vi "Merge Sort Transposed Time Series Data.vi"(0 "Time Series Array A":dbl[][](array[numeric]), 1 "Ignore Duplicates? (F)":bool, 3 "Time Series Array B":dbl[][](array[numeric])) -> (6 "Sorted Time Series Array":dbl[][](array[numeric]))   [LabVIEW 2013, in "Data Log Fetcher.lvlib"]
uses:
  Data Log Fetcher.lvlib
panel:
  out "A Index":i32
  out "B Index":i32
  out "B Count":i32
  out "A Count":i32
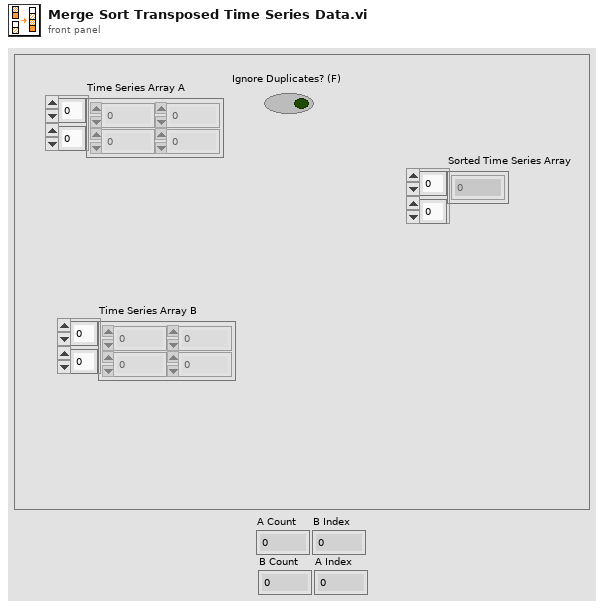
[diagram p1: front panel]
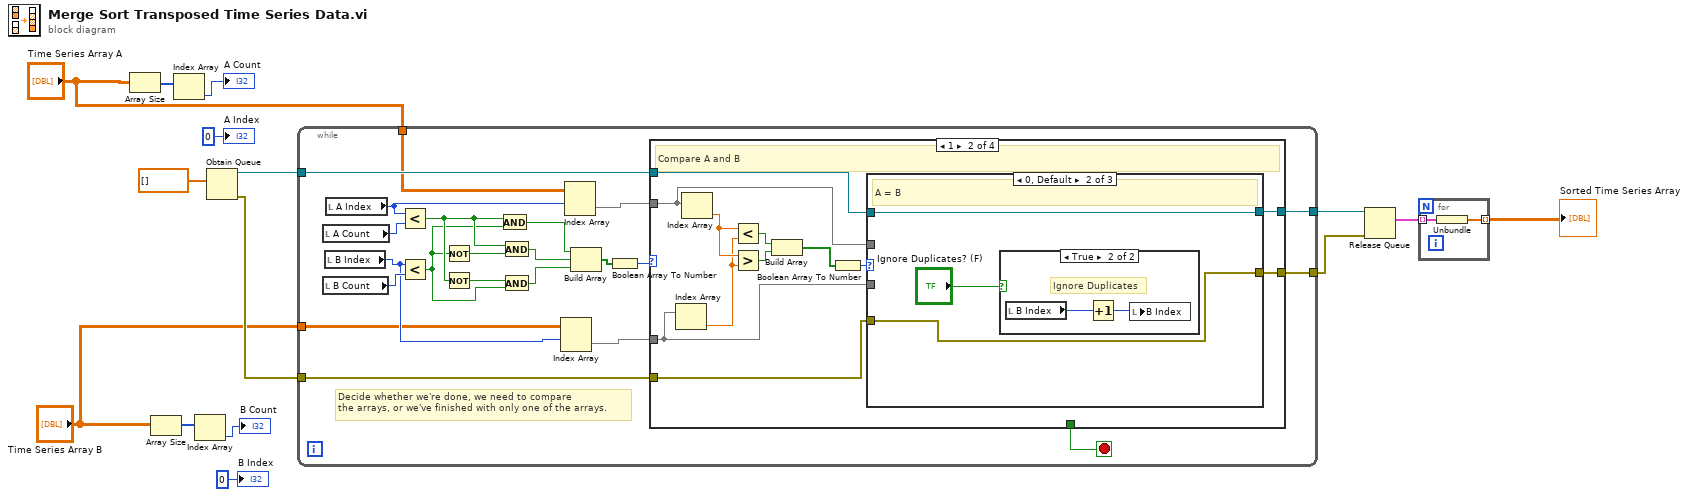
[diagram p0: block diagram]
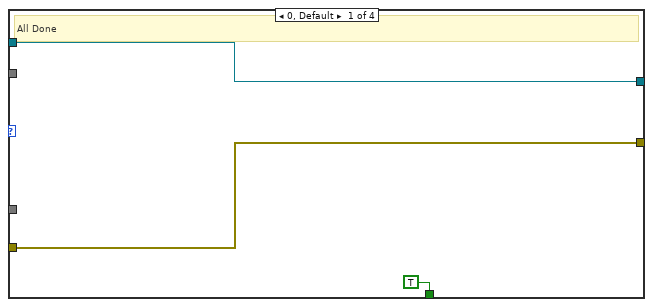
[diagram p2: hidden frame]
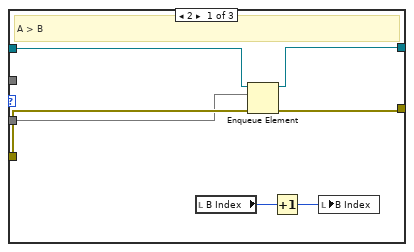
[diagram p3: hidden frame]
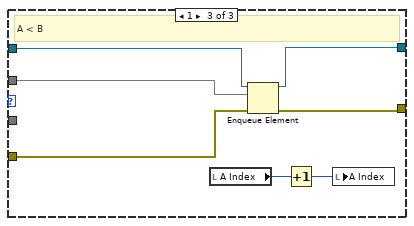
[diagram p5: hidden frame]
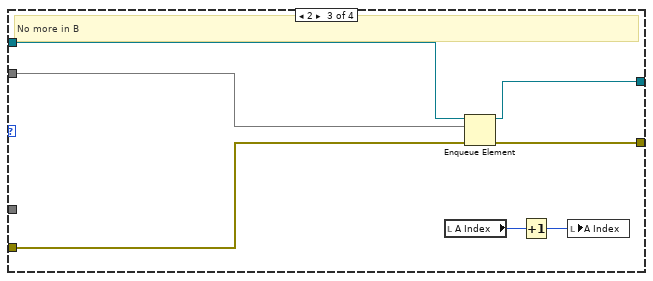
[diagram p6: hidden frame]
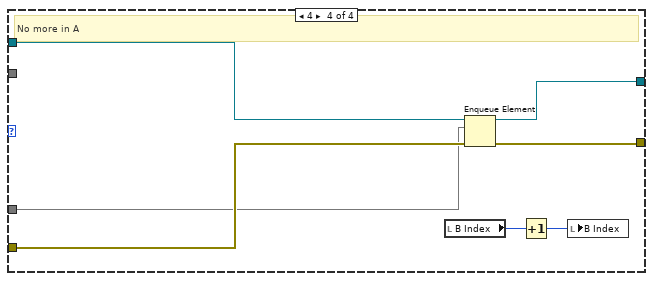
[diagram p7: hidden frame]
diagram:
  n1 = Array Size(array="Time Series Array A") -> (size(s)=w8:i32[])
  n2 = Array Size(array="Time Series Array B") -> (size(s)=w6:i32[])
  n3 = Index Array(array=w8) -> (element=→"A Count":i32)  [unwired: 1 in]
  n4 = Index Array(array=w6) -> (element=→"B Count":i32)  [unwired: 1 in]
  n5 = Obtain Queue(element data type=dbl[] []) -> (queue out=w14:refnum<queue>, error out=w13:errorcluster)  [unwired: 4 in, 1 out]
  n6 = while {
    tunnel: w14 -> [w26]
    tunnel: [w25] -> w10
    tunnel: [w24] -> w15
    tunnel: w13 -> [w23]
    tunnel: "Time Series Array A" -> [w17]
    tunnel: "Time Series Array B" -> [w16]
    stop <- w18 stop-if-true
    # "Decide whether we're done, we need to compare\nthe arrays, or we've finished with only one of the arrays."
    n7 = local read "A Count"() -> (w37:i32)
    n8 = local read "B Count"() -> (w36:i32)
    n9 = local read "B Index"() -> (w21:i32)
    n10 = local read "A Index"() -> (w22:i32)
    n11 = Less?(x=w22, y=w37) -> (x < y?=w33:bool)
    n12 = Less?(x=w21, y=w36) -> (x < y?=w32:bool)
    n13 = Not(x=w32) -> (.not. x?=w30:bool)
    n14 = Not(x=w33) -> (.not. x?=w29:bool)
    n15 = And(x=w33, y=w32) -> (x .and. y?=w35:bool)
    n16 = And(x=w33, y=w30) -> (x .and. y?=w34:bool)
    n17 = And(x=w29, y=w32) -> (x .and. y?=w31:bool)
    n18 = Index Array(array=w16, index (row)=w21) -> (element=w20:dbl[])  [unwired: 1 in]
    n19 = Index Array(array=w17, index (row)=w22) -> (element=w19:dbl[])  [unwired: 1 in]
    n20 = Build Array(w35, w34, w31) -> (w28:bool[])
    n21 = Boolean Array To Number(Boolean array=w28) -> (number=w27:u32)
    n22 = case shown="1" w27 {
      tunnel: w26 -> [w40 w52 w78 w85]
      tunnel: w19 -> [_ w44 w76 _]
      tunnel: w20 -> [_ w42 _ w83]
      tunnel: w23 -> [w39 w45 w77 w84]
      tunnel: [w39 w51 w74 w81] -> w25
      tunnel: [w40 w50 w75 w82] -> w24
      tunnel: [TRUE _ _ _] -> w18
      frame 0, Default {
        # "All Done"
      }
      frame 1 {
        # "Compare A and B"
        n23 = Index Array(array=w42) -> (element=w41:dbl)  [unwired: 1 in]
        n24 = Index Array(array=w44) -> (element=w43:dbl)  [unwired: 1 in]
        n25 = Less?(x=w43, y=w41) -> (x < y?=w49:bool)
        n26 = Greater?(x=w43, y=w41) -> (0:w48:bool)
        n27 = Build Array(w49, w48) -> (w47:bool[])
        n28 = Boolean Array To Number(Boolean array=w47) -> (number=w46:u32)
        n29 = case shown="0, Default" w46 {
          tunnel: w52 -> [w59 w60 w71]
          tunnel: w44 -> [_ _ w70]
          tunnel: w42 -> [w53 _ _]
          tunnel: w45 -> [w58 w61 w69]
          tunnel: [w56 w61 w67] -> w51
          tunnel: [w57 w60 w68] -> w50
          frame 2 {
            # "A > B"
            n30 = local read "B Index"() -> (w54:i32)
            n31 = Enqueue Element(queue=w59, element=w53, error in (no error)=w58) -> (queue out=w57:refnum<queue>, error out=w56:errorcluster)  [unwired: 1 in, 1 out]
            n32 = Increment(x=w54) -> (x+1=w55:i32)
            n33 = local write "B Index"(w55) -> ()
          }
          frame 0, Default {
            # "A = B"
            n34 = case shown="True" "Ignore Duplicates? (F)" {
              frame False {
              }
              frame True {
                # "Ignore Duplicates"
                n35 = local read "B Index"() -> (w64:i32)
                n36 = Increment(x=w64) -> (x+1=w63:i32)
                n37 = local write "B Index"(w63) -> ()
              }
            }
          }
          frame 1 {
            # "A < B"
            n38 = local read "A Index"() -> (w65:i32)
            n39 = Enqueue Element(queue=w71, element=w70, error in (no error)=w69) -> (queue out=w68:refnum<queue>, error out=w67:errorcluster)  [unwired: 1 in, 1 out]
            n40 = Increment(x=w65) -> (x+1=w66:i32)
            n41 = local write "A Index"(w66) -> ()
          }
        }
      }
      frame 2 {
        # "No more in B"
        n42 = local read "A Index"() -> (w72:i32)
        n43 = Enqueue Element(queue=w78, element=w76, error in (no error)=w77) -> (queue out=w75:refnum<queue>, error out=w74:errorcluster)  [unwired: 1 in, 1 out]
        n44 = Increment(x=w72) -> (x+1=w73:i32)
        n45 = local write "A Index"(w73) -> ()
      }
      frame 4 {
        # "No more in A"
        n46 = local read "B Index"() -> (w79:i32)
        n47 = Enqueue Element(queue=w85, element=w83, error in (no error)=w84) -> (queue out=w82:refnum<queue>, error out=w81:errorcluster)  [unwired: 1 in, 1 out]
        n48 = Increment(x=w79) -> (x+1=w80:i32)
        n49 = local write "B Index"(w80) -> ()
      }
    }
  }
  n50 = Release Queue(queue=w15, error in (no error)=w10) -> (remaining elements=w4:cluster{dbl[]}[])  [unwired: 1 in, 2 out]
  n51 = for {
    tunnel: w4 -> [w87] mode=indexing
    tunnel: [w86] -> w3 mode=indexing
    n52 = Unbundle(w87) -> (w86:dbl[])
  }
  "Sorted Time Series Array" <- w3
  "A Index" <- 0 ("A Index")
  "B Index" <- 0 ("B Index")
